vi "Counter - Read Encoder.vi"() -> ()   [LabVIEW 2017]
doc: "本范例演示用一个计数器连续监控编码器角位置的方法。\n\n关于将信号连接至DAQ设备的方法，可参考设备文档。"
uses:
  <vilib>/Utility/error.llb/DialogType.ctl
  <vilib>/DAQmx/read.llb/DAQmx Read (Counter DBL 1Chan 1Samp).vi
  <vilib>/DAQmx/create/channels.llb/DAQmx Create Channel (CI-Position-Angular Encoder).vi
  <vilib>/DAQmx/miscellaneous.llb/DAQmx Fill In Error Info.vi
  <resource>/objmgr/daqmx.rc
panel:
  in  "Z索引接线端":tag="PFI9"
  in  "启用Z索引":bool
  in  "脉冲每转":u32=24
  in  "B输入接线端":tag="PFI10"
  out "位置":dbl
  in  "输入接线端":tag="PFI8"
  in  "计数器":tag="Dev1/ctr0"
  in  "触发类型":enum32{"No Trigger", "Digital Arm Start"}(tab)
  in  "边沿":i32(ring)=10280 items=["上升"=10280, "下降"=10171]
  in  "数字触发源":tag
  in  "停止":bool
  in  "循环时间(ms)":u32=10
  # "通道设置"
  # "采集数据"
  # "定时设置"
  # "触发设置"
  # "如需配置并使用触发/计数重置，必须先在上面选择相应的选项卡。  有些硬件不支持上述选项－更多信息见设备的相应文档。"
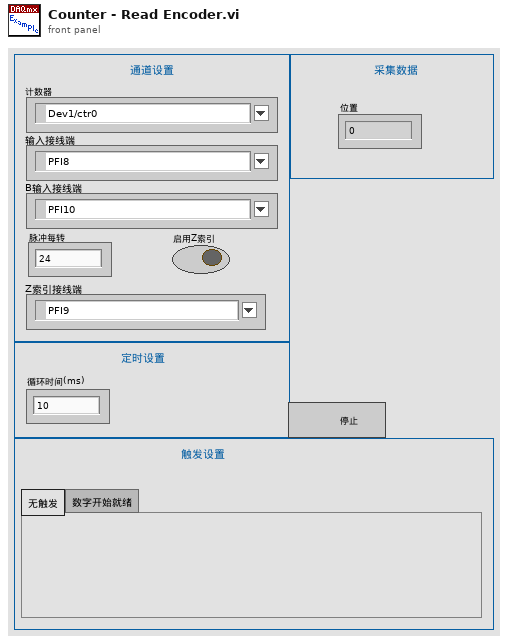
[diagram p1: front panel]
types:
  T1 = typedef "DialogType.ctl" = u16
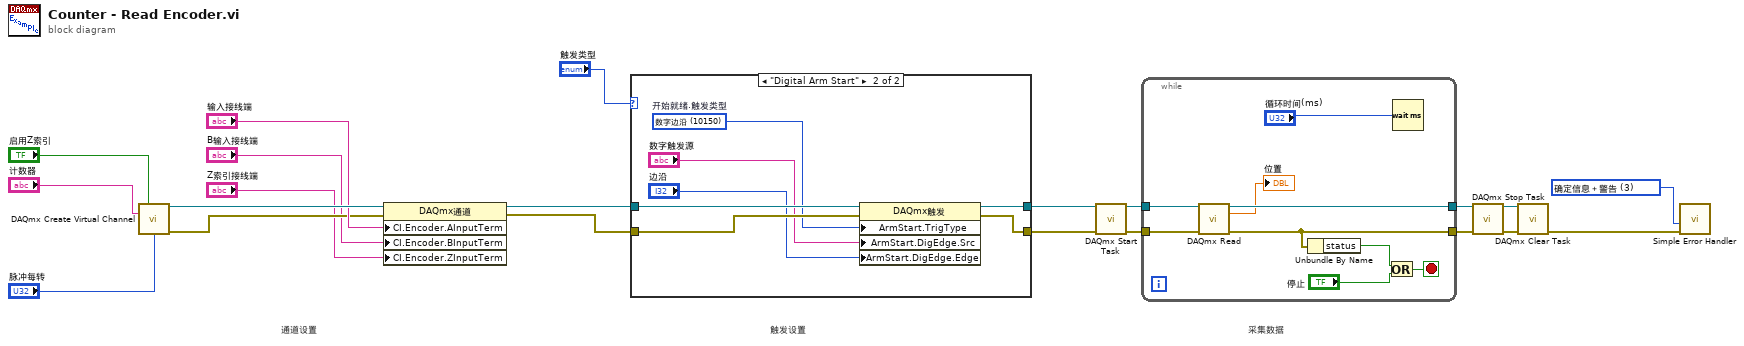
[diagram p0: block diagram]
diagram:
  w1 = T1 3 items=["无对话框", "确定信息", "继续或停止信息", "确定信息＋警告", "继续/停止＋警告"] ("对话框类型（确定信息：1）")
  # "采集数据"
  # "触发设置"
  # "通道设置"
  n1 = call-poly <vilib>:"DAQmx Create Virtual Channel.vi"("z index enable"="启用Z索引", "counter"="计数器", "pulses per revolution"="脉冲每转") -> ("task out"=w14:refnum<k21>, "error out"=w12:errorcluster)  [unwired: 11 in]
  n2 = property class="DAQmx通道"(reference=w14, error in=w12, "CI.Encoder.AInputTerm"="输入接线端", "CI.Encoder.BInputTerm"="B输入接线端", "CI.Encoder.ZInputTerm"="Z索引接线端") -> (reference out=w10:refnum<k21>, error out=w11:errorcluster)
  n3 = case shown="\"Digital Arm Start\"" "触发类型" {
    tunnel: w10 -> [w23 w30]
    tunnel: w11 -> [w22 w27]
    tunnel: [w23 w29] -> w21
    tunnel: [w22 w28] -> w20
    frame "No Trigger", Default {
    }
    frame "Digital Arm Start" {
      w24 = 10150 items=["数字边沿"=10150, "无"=10230]  # 开始就绪.触发类型
      n4 = property class="DAQmx触发"(reference=w30, error in=w27, "ArmStart.TrigType"=w24, "ArmStart.DigEdge.Src"="数字触发源", "ArmStart.DigEdge.Edge"="边沿") -> (reference out=w29:refnum<k21>, error out=w28:errorcluster)
    }
  }
  n5 = call <vilib>:"DAQmx Start Task.vi"("task/channels in"=w21, "error in"=w20) -> ("task out"=w19:refnum<k21>, "error out"=w18:errorcluster)  [unwired: 12 in]
  n6 = while {
    tunnel: w19 -> [w39]
    tunnel: w18 -> [w38]
    tunnel: [w35] -> w4
    tunnel: [w36] -> w5
    stop <- w37 stop-if-true
    n7 = call-poly <vilib>:"DAQmx Read.vi"("task/channels in"=w39, "error in"=w38) -> ("task out"=w36:refnum<k21>, "data"=→"位置":dbl, "error out"=w35:errorcluster)  [unwired: 11 in]
    n8 = Unbundle By Name(w35) -> ("status"=w34:bool)
    n9 = Or(x=w34, y="停止") -> (x .or. y?=w37:bool)
    n10 = Wait (ms)(milliseconds to wait="循环时间(ms)") -> ()  [unwired: 1 out]
  }
  n11 = call <vilib>:"DAQmx Stop Task.vi"("task/channels in"=w5, "error in"=w4) -> ("task out"=w2:refnum<k21>, "error out"=w3:errorcluster)  [unwired: 12 in]
  n12 = call <vilib>:"DAQmx Clear Task.vi"("task in"=w2, "error in"=w3) -> ("error out"=w17:errorcluster)  [unwired: 13 in]
  n13 = call <vilib>:"Simple Error Handler.vi"("type of dialog (OK msg:1)"=w1, "error in (no error)"=w17) -> ()  [unwired: 3 in, 5 out]
